vi "VdTcpIP_Create.vi"(0 "reference":refnum<class "VdTcpIP.lvclass">, 1 "IP-Address":string, 2 "Port":u16, 3 "Connection":refnum<k5>, 4 "OnNewConnectionRunThisVI(Path or Name)":variant, 5 "error in (no error)":errorcluster, 6 "OnlyCreateOneObjectFor_<Ip-Address/Port>_Combination(False)":bool, 7 "DataToNewConnectionVI":T1(array[cluster])) -> (14 "reference out":refnum<class "VdTcpIP.lvclass">, 17 "ObjectCreated":bool, 19 "error out":errorcluster)   [LabVIEW 2020, in "VdTcpIP.lvclass"]
doc: "Creates and initializes a new VdSocket object.\nIf the input <B>IP-Address</B> is left empty, this object will be a TCP/IP listener."
uses:
  VdTcpIP.lvclass
panel:
  # "The input reference should only\nbe wired when this method is called\nby a sub class constructor."
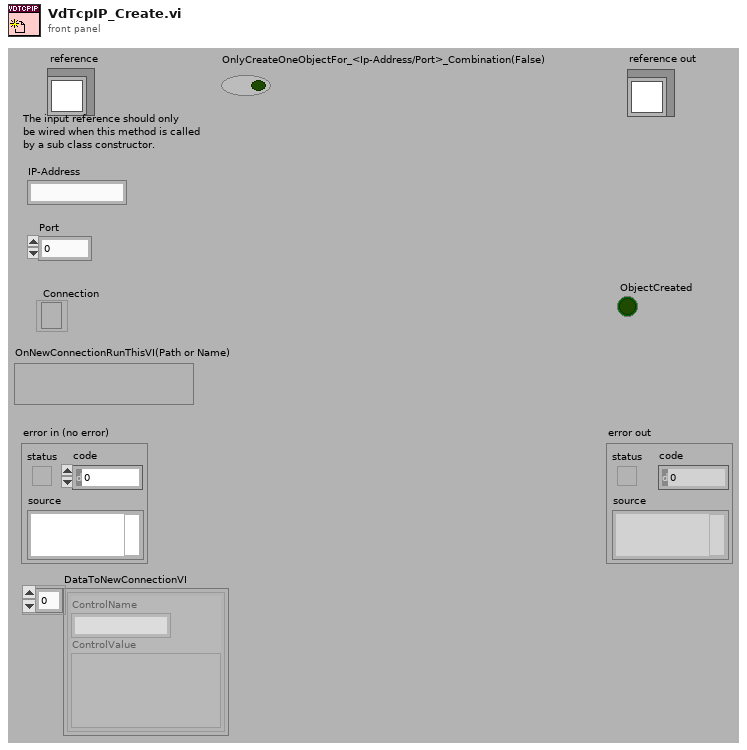
[diagram p1: front panel]
types:
  T1 = cluster{"ControlName":string, "ControlValue":variant}[]
  T2 = enum16{"Create or look up existing", "Look up existing"}
  T3 = typedef "Semaphore RefNum" = refnum<k1>
  T4 = typedef "VdTcpIP.lvclass/ObjectAttributes.ctl" = cluster{"IP-Address":string, "Port":u16, "Connection":refnum<k5>, "Listener":refnum<k5>, "ListenerConnection":refnum<k5>, "Listner":bool, "ListnerProcessRunning":bool, "InConnections":refnum<k5>[], "InConnectionsIP":string[], "InConnectionAdded":refnum<notifier>, "RunVIOnNewConnection":variant, "DataToNewConnectionVI":cluster{"ControlName":string, "ControlValue":variant}[], "WebServicesURL_Location(http://...)":string, "WebServicesPostWebPage(*.asmx)":string, "Semaphore":T3, "AutoReConnectTimes":i32, "AutoReConnectInterval(ms)":i32, "ConnectionTimeout":i32}
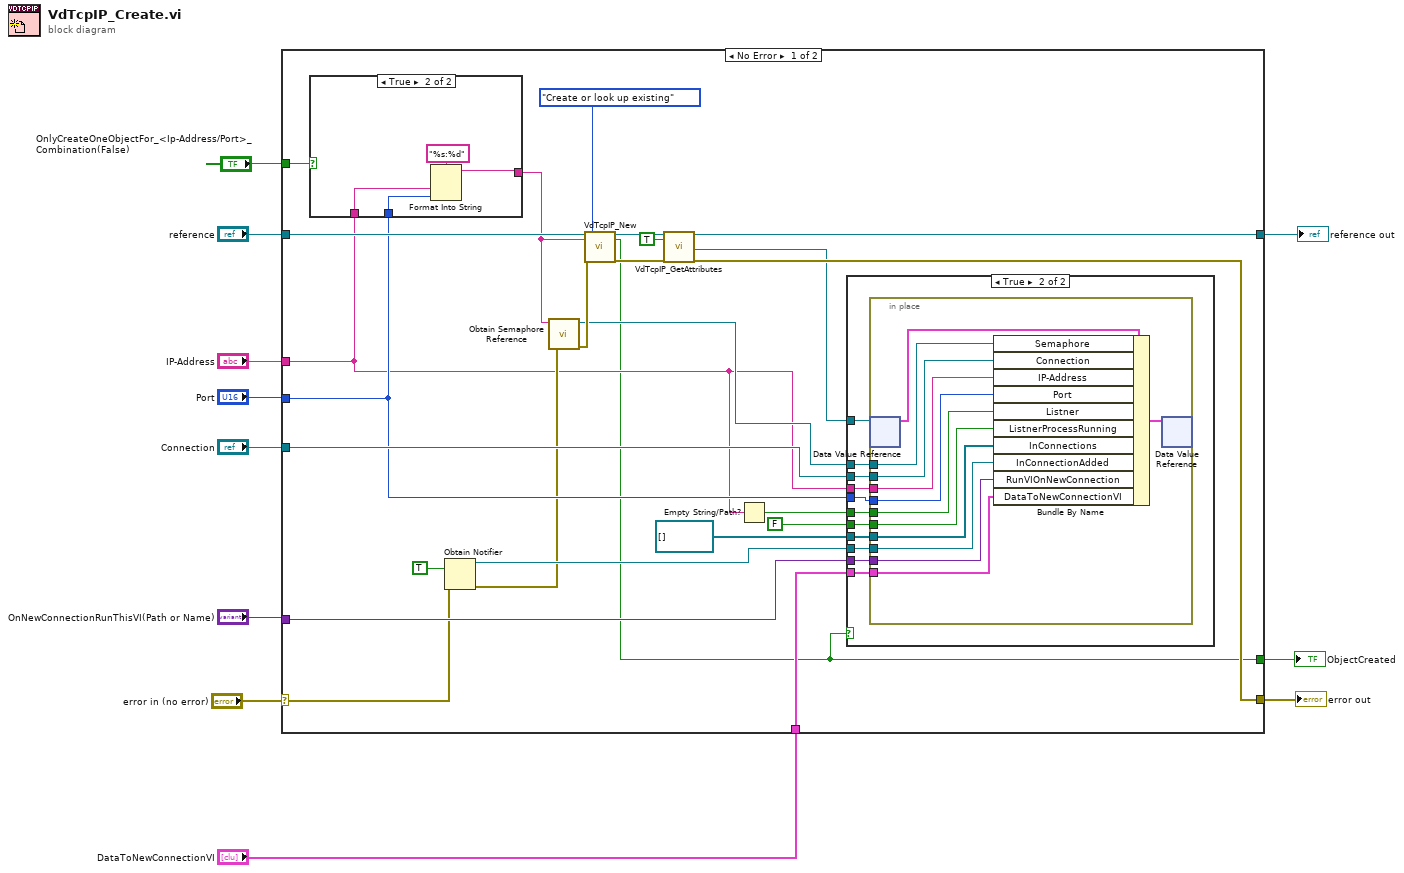
[diagram p0: block diagram]
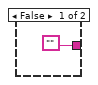
[diagram p3: hidden frame]
diagram:
  n1 = case shown="No Error" "error in (no error)" {
    selector: "error in (no error)" -> [w14 w66]
    tunnel: [w34 w65] -> w11
    tunnel: [w36 w66] -> w10
    tunnel: "reference" -> [w33 w65]
    tunnel: "IP-Address" -> [w13 _]
    tunnel: "Port" -> [w23 _]
    tunnel: "Connection" -> [w24 _]
    tunnel: "OnNewConnectionRunThisVI(Path or Name)" -> [w18 _]
    tunnel: "DataToNewConnectionVI" -> [w17 _]
    tunnel: "OnlyCreateOneObjectFor_<Ip-Address/Port>_Combination(False)" -> [w30 _]
    tunnel: [w12 _] -> w1
    frame No Error {
      n2 = case shown="True" w30 {
        tunnel: ["" w61] -> w28
        tunnel: w13 -> [_ w64]
        tunnel: w23 -> [_ w62]
        frame False {
        }
        frame True {
          n3 = Format Into String(format string="%s:%d", w64, w62) -> (resulting string=w61:string)  [unwired: 2 in, 1 out]
        }
      }
      n4 = Obtain Notifier(notification data type=TRUE, error in (no error)=w14) -> (notifier out=w19:refnum<notifier>, error out=w15:errorcluster)  [unwired: 1 in, 2 out]
      n5 = call <vilib>:"Obtain Semaphore Reference.vi"("error in (no error)"=w15, "name (unnamed)"=w28) -> ("error out"=w29:errorcluster, "semaphore"=w25:T3)  [unwired: 3 in, 1 out]
      n6 = call "VdTcpIP_New.vi"("reference in"=w33, "Object name"=w28, "error in (no error)"=w29, "CreateMethod(Create or look up existing)"=T2."Create or look up existing" ("Create method")) -> ("reference out"=w35:refnum<class "VdTcpIP.lvclass">, "NewObjectCreated"=w12:bool, "error out"=w31:errorcluster)  [unwired: 13 out]
      n7 = call "VdTcpIP_GetAttributes.vi"("reference in"=w35, "OnlyGetDvrReference(False)"=TRUE, "error in (no error)"=w31) -> ("reference out"=w34:refnum<class "VdTcpIP.lvclass">, "DataRef"=w26:refnum<data-value>, "error out"=w36:errorcluster)  [unwired: 13 in, 1 out]
      n8 = Empty String/Path?(string/path=w13) -> (empty?=w22:bool)
      n9 = case shown="True" w12 {
        tunnel: w26 -> [_ w47]
        tunnel: w25 -> [_ w46]
        tunnel: w24 -> [_ w45]
        tunnel: w23 -> [_ w44]
        tunnel: w22 -> [_ w43]
        tunnel: FALSE ("ListnerProcessRunning") -> [_ w42]
        tunnel: refnum<k5>[] [] ("EmptyConnection") -> [_ w41]
        tunnel: w19 -> [_ w40]
        tunnel: w18 -> [_ w39]
        tunnel: w17 -> [_ w38]
        tunnel: w13 -> [_ w37]
        frame False {
        }
        frame True {
          n10 = in-place {
            in-place-border: w46 -> [w58]
            in-place-border: w45 -> [w57]
            in-place-border: w37 -> [w56]
            in-place-border: w44 -> [w55]
            in-place-border: w43 -> [w54]
            in-place-border: w42 -> [w53]
            in-place-border: w41 -> [w52]
            in-place-border: w40 -> [w51]
            in-place-border: w39 -> [w50]
            in-place-border: w38 -> [w49]
            n11 = in-place-dvr #1(w47) -> (w59:T4)  [unwired: 1 out]
            n12 = Bundle By Name(cluster=w59, "Semaphore"=w58, "Connection"=w57, "IP-Address"=w56, "Port"=w55, "Listner"=w54, "ListnerProcessRunning"=w53, "InConnections"=w52, "InConnectionAdded"=w51, "RunVIOnNewConnection"=w50, "DataToNewConnectionVI"=w49) -> (w48:T4)
            n13 = in-place-dvr #1(w48) -> ()  [unwired: 2 out]
          }
        }
      }
    }
    frame Error {
    }
  }
  "error out" <- w10
  "reference out" <- w11
  "ObjectCreated" <- w1
